vi "modbusRxLoop.vi"(11 "Modbus Port Settings":T1={"Tx Port"="ModbusPort1Tx", "Tx Data FIFO"="txModbusPort1FIFO", "Tx Internal FIFO"="txModbusPort1InternalFIFO", "Tx Telemetry FIFO"="txModbusPort1TelemetryFIFO", "Rx Port"="ModbusPort1Rx", "Rx Data FIFO"="rxModbusPort1FIFO", "Rx Telemetry FIFO"="txModbusPort1TelemetryFIFO", "Base Telemetry Address"=0, "Wait For Rx Frame Register"="WaitForPort1RxFrame", "IRQ Address"=0, "Trigger IRQ Register"="TriggerPort1IRQ", "Trigger IRQ Response Register"="TriggerPort1IRQ"}) -> ()   [LabVIEW 2015]
uses:
  DataTypes/ModbusPortSettings.ctl
  DataTypes/RxLoopData.ctl
  DataTypes/RxStates.ctl
  <vilib>/Platform/TimedLoop/XDataNode/timing_clust.ctl
  <vilib>/Platform/TimedLoop/XDataNode/nitl_modes.ctl
  <vilib>/Platform/TimedLoop/XDataNode/wakeup.ctl
  Telemetry/DataTypes/TelemetryUpdateMode.ctl
  <vilib>/rvi/Emulation/niFpgaSctlEmulationGetInTimedLoop.vi
  <vilib>/rvi/Emulation/niFpgaEmulationReportErrorSimple.vi
  <vilib>/rvi/Emulation/niFpgaGetClockAttributes.vi
  <vilib>/rvi/Emulation/niFpgaCriticalErrorInLSC.vi
  <vilib>/rvi/Emulation/niFpgaEmulationIsFPGAContextNoSignature.vi
  <vilib>/rvi/DataTransferAndStorage/Container/Common/niFpgaContainerGetUniqueNameForEmu.vi
  <vilib>/rvi/Memory/Memory_Emulation/niFpgaMemoryEmulationCacheClearOnFirstRun.vi
  <vilib>/rvi/Memory/Memory_Emulation/nirvimemoryEmulationManagerCache_MakeExclusive.vi
  <vilib>/rvi/Memory/Memory_Emulation/niFpgaMemoryEmulationValidateCache.vi
  <vilib>/rvi/Memory/Memory_Emulation/nirvimemoryEmulationManagerCache_InsertValue.vi
  <vilib>/Utility/error.llb/Clear Errors.vi
  <vilib>/rvi/Memory/Memory_Emulation/nirvimemoryEmulationManagerCache_ReleaseExclusive.vi
  <vilib>/rvi/Memory/Memory_Emulation/nirvimemoryEmulationManagerCache_GetValue.vi
  <vilib>/rvi/Memory/Memory_Emulation/nirvimemoryEmulationManagerCache_SetValue.vi
  <vilib>/rvi/Emulation/niFpgaProcessEmulError.vi
  <vilib>/rvi/eio/common/nirviEmuTemplateMethod_errors.vi
  <vilib>/rvi/DataTransferAndStorage/Container/Common/niFpgaContainerExecOnDevCompGetState.vi
  <vilib>/rvi/errors/niFpgaSetErrorForExecOnDevCompSimple.vi
  <vilib>/rvi/eio/common/nirviEmuReportErrorAndStop.vi
  <vilib>/rvi/FIFO/Fifo_Resource/nirvififoEmulationSetSize.vi
  <vilib>/rvi/FIFO/Fifo_Resource/nirviFifoEmulationQueueMgr.vi
  <instcachedir>/0/nirviFifoEmulationQueueMgr_E5CAEC123FF24DC58D834DCA3CDAA9B5.lvgen/nirviFifoEmulationQueueMgr_E5CAEC123FF24DC58D834DCA3CDAA9B5_005.vi
  <vilib>/rvi/FIFO/Fifo_Resource/nirvififoEmulationDetermineInputValidOut.vi
  <vilib>/rvi/FIFO/Fifo_Resource/nirvififoEmulationCreateLock.vi
  <vilib>/rvi/FIFO/Fifo_Resource/nirvififoEmulationObtainLock.vi
  <vilib>/rvi/FIFO/Fifo_Resource/nirvififoEmulationReleaseLock.vi
  <vilib>/rvi/occurrence/nirviWaitOnOccurrenceBase.vi
  <vilib>/rvi/errors/nirviReportUnexpectedCaseInternalError.vi
  <vilib>/rvi/errors/nirviReportUnexpectedCaseInternalError (U32).vi
  <vilib>/rvi/interface/RandomDataEmulation/niFpgaRandomDataHandleErrors.vi
  <vilib>/Platform/TimedLoop/XDataNode/XDataNode.xnode
  <vilib>/rvi/DataTransferAndStorage/Container/XNode/niFpgaContainer.xnode
  <vilib>/rvi/DataTransferAndStorage/Register/Emulation/niFpgaRegisterEmulation.vi
  <vilib>/eio/EIONode/EIONode.xnode
  <vilib>/rvi/FIFO/Fifo_Resource/niFpgaFifoEmulationRefIn.vi
  <vilib>/rvi/DataTransferAndStorage/Register/Emulation/niFpgaRegisterEmulationRefIn.vi
  <vilib>/Platform/TimedLoop/XDataNode/XDNodeRunTimeDep.lvlib
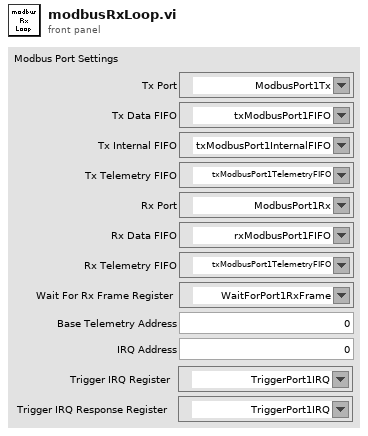
[diagram p1: front panel]
types:
  T1 = typedef "ModbusPortSettings.ctl" = cluster{"Tx Port":refnum<k21>, "Tx Data FIFO":refnum<k21>, "Tx Internal FIFO":refnum<k21>, "Tx Telemetry FIFO":refnum<k21>, "Rx Port":refnum<k21>, "Rx Data FIFO":refnum<k21>, "Rx Telemetry FIFO":refnum<k21>, "Base Telemetry Address":u32, "Wait For Rx Frame Register":refnum<k21>, "IRQ Address":u8, "Trigger IRQ Register":refnum<k21>, "Trigger IRQ Response Register":refnum<k21>}
  T2 = typedef "RxLoopData.ctl" = cluster{"State":T3, "Delay Ticks":u16, "State After Delay":T3, "Number of Samples":u16, "Sample":u8, "Data":u16, "Bits":u16, "State After Insert Sample":T3, "Received Data":bool, "Enqueue Data Time":u32, "Previous Level":bool}
  T3 = typedef "RxStates.ctl" = enum16{"WaitForFallingEdge", "Delay", "SampleStartBit", "SampleBit", "EnqueueData", "EnqueueEndOfFrame"}
  T4 = typedef "XDNodeRunTimeDep.lvlib/timing_clust.ctl" = cluster{"Expected End [f-1]":u64, "Actual End [f-1]":u64, "Finished Late? [f-1]":bool, "Expected End [i-1]":u64, "Actual End [i-1]":u64, "Finished Late? [i-1]":bool, "Expected Start [i]":u64, "Actual Start [i]":u64, "Expected Start [f]":u64, "Actual Start [f]":u64, "Source Name":string, "Structure Name":string, "Period":i64, "Deadline":i64, "Offset":i64, "Start":i64, "Priority":i32, "Timeout":i32, "Mode":T5, "Wakeup Reason":T6, "Error":errorcluster, "Source Type":string, "Secondary Source Type":string, "Global End Time":u64, "Global Start Time":u64, "Frame Duration":u64, "Iteration Duration":u64, "Assigned CPU":i32, "I/O Scan Engine Mode":u32}
  T5 = typedef "XDNodeRunTimeDep.lvlib/nitl_modes.ctl" = enum32{"No Change", "Process missed periods, maintain original phase", "Discard missed periods, maintain original phase", "Process missed periods, ignore original phase", "Discard missed periods, ignore original phase"}
  T6 = typedef "XDNodeRunTimeDep.lvlib/wakeup.ctl" = enum32{"Normal", "Aborted", "Asynchronous wakeup", "Timing source error", "Timed loop error", "Timeout"}
  T7 = typedef "TelemetryUpdateMode.ctl" = enum8{"NOP", "Set", "Add", "Subtract", "Or"}
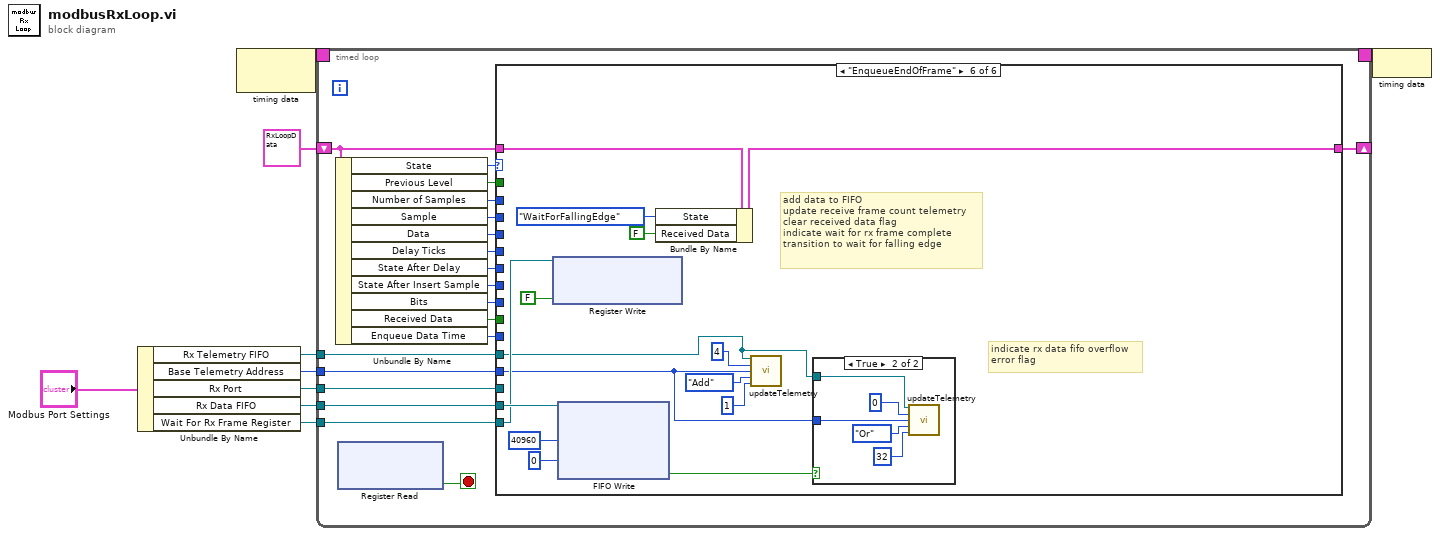
[diagram p0: block diagram]
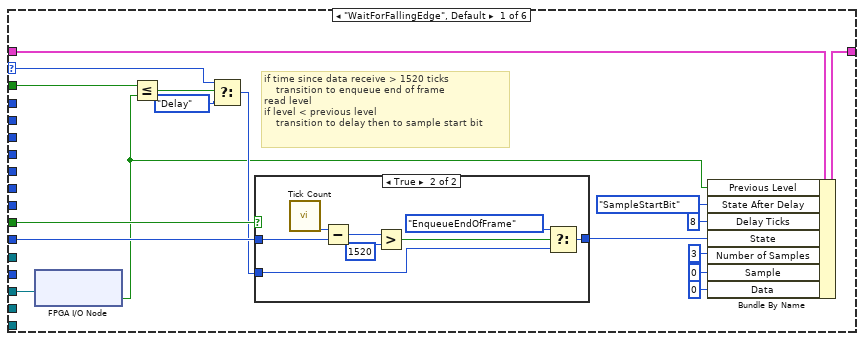
[diagram p2: hidden frame]
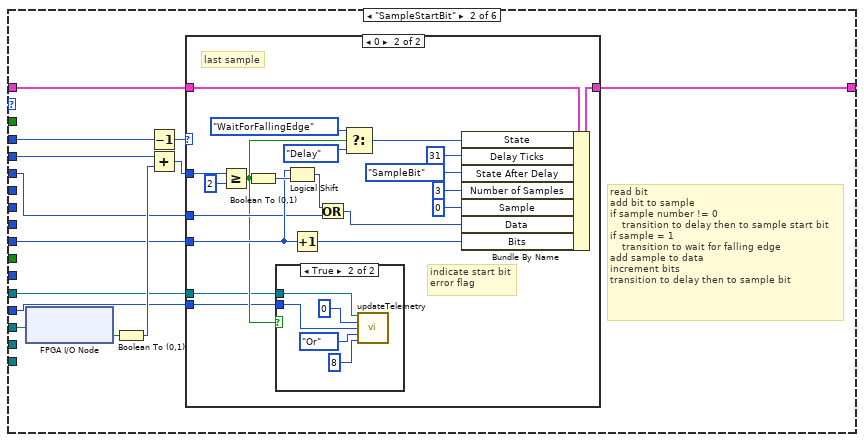
[diagram p4: hidden frame]
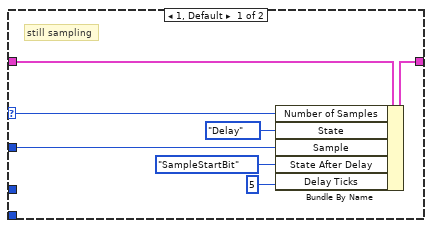
[diagram p5: hidden frame]
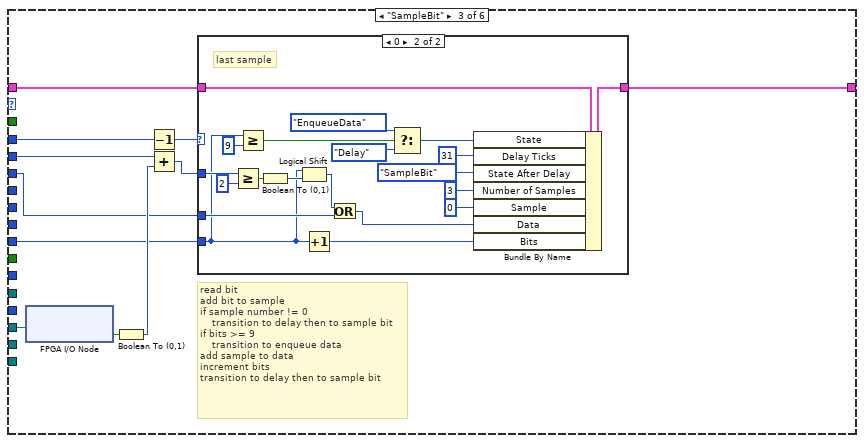
[diagram p7: hidden frame]
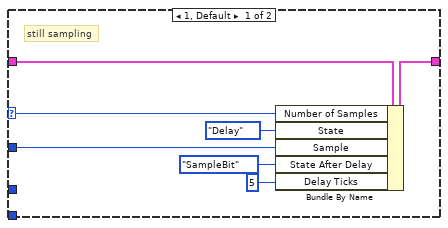
[diagram p8: hidden frame]
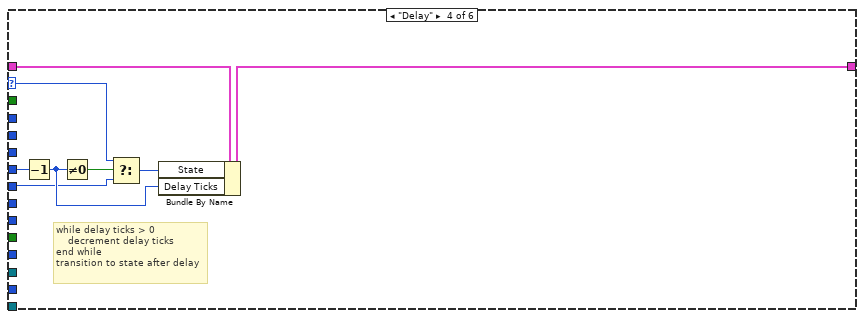
[diagram p9: hidden frame]
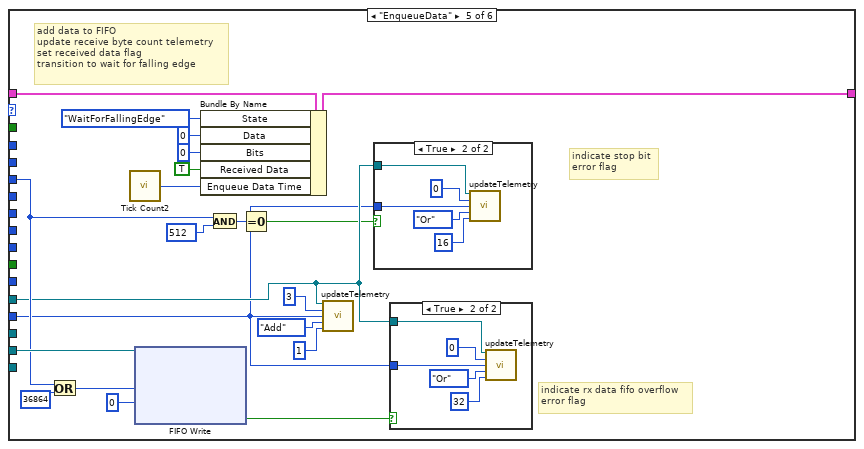
[diagram p10: hidden frame]
diagram:
  n1 = Unbundle By Name("Modbus Port Settings") -> ("Rx Telemetry FIFO"=w6:refnum<k21>, "Base Telemetry Address"=w3:u32, "Rx Port"=w4:refnum<k21>, "Rx Data FIFO"=w5:refnum<k21>, "Wait For Rx Frame Register"=w7:refnum<k21>)
  n2 = node-c288() -> (w9:T4)  [unwired: 1 in]
  n3 = timed-loop {
    tunnel: w4 -> [w25]
    tunnel: w5 -> [w16]
    shift-right: [w24] -> _
    shift-left: T2 {"State"=enum."WaitForFallingEdge", "Delay Ticks"=0, "State After Delay"=enum."WaitForFallingEdge", "Number of Samples"=0, "Sample"=0, "Data"=0, "Bits"=0, "State After Insert Sample"=enum."WaitForFallingEdge", "Received Data"=FALSE, "Enqueue Data Time"=0, "Previous Level"=FALSE} ("ModbusRxLoop") -> [w27]
    tunnel: w3 -> [w13]
    timing: w9 -> [_]
    timing-out: [_] -> w8
    tunnel: w6 -> [w11]
    tunnel: w7 -> [w10]
    stop <- w28 stop-if-true
    n4 = Unbundle By Name(w27) -> ("State"=w26:T3, "Previous Level"=w12:bool, "Number of Samples"=w23:u16, "Sample"=w22:u8, "Data"=w21:u16, "Delay Ticks"=w20:u16, "State After Delay"=w19:T3, "State After Insert Sample"=w18:T3, "Bits"=w17:u16, "Received Data"=w14:bool, "Enqueue Data Time"=w15:u32)
    n5 = xnode ("Register Read")() -> ("Data"=w28:bool)  [unwired: 1 in, 1 out]
    n6 = case shown="\"EnqueueEndOfFrame\"" w26 {
      selector: w26 -> [w44 _ _ w142 _ _]
      tunnel: w27 -> [w38 w62 w105 w139 w165 w188]
      tunnel: w25 -> [w45 w66 w109 _ _ _]
      tunnel: [w41 w61 w104 w138 w164 w185] -> w24
      tunnel: w23 -> [_ w67 w110 _ _ _]
      tunnel: w22 -> [_ w64 w107 _ _ _]
      tunnel: w21 -> [_ w57 w100 _ w151 _]
      tunnel: w20 -> [_ _ _ w140 _ _]
      tunnel: w19 -> [_ _ _ w141 _ _]
      tunnel: w18 -> [_ _ _ _ _ _]
      tunnel: w17 -> [_ w58 w101 _ _ _]
      tunnel: w16 -> [_ _ _ _ w166 w191]
      tunnel: w15 -> [w43 _ _ _ _ _]
      tunnel: w14 -> [w42 _ _ _ _ _]
      tunnel: w13 -> [_ w55 _ _ w147 w179]
      tunnel: w12 -> [w32 _ _ _ _ _]
      tunnel: w11 -> [_ w56 _ _ w148 w178]
      tunnel: w10 -> [_ _ _ _ _ w180]
      frame "WaitForFallingEdge", Default {
        # "if time since data receive > 1520 ticks\n    transition to enqueue end of frame\nread level\nif level < previous level\n    transition to delay then to sample start bit"
        n7 = xnode "FPGA I/O Node"("FPGA I/O In"=w45) -> ("I/O Item"=w29:bool)  [unwired: 1 out]
        n8 = Less Or Equal?(x=w32, y=w29) -> (x <= y?=w35:bool)
        n9 = Select(t=w44, s=w35, f=RxStates."Delay" ("State After Delay")) -> (s? t:f=w34:T3)
        n10 = case shown="True" w42 {
          tunnel: w43 -> [_ w53]
          tunnel: w34 -> [w46 w48]
          tunnel: [w46 w47] -> w39
          frame False {
          }
          frame True {
            n11 = call "Tick Count"() -> ("Tick Count(Ticks)"=w54:u32)
            n12 = Subtract(x=w54, y=w53) -> (x-y=w52:u32)
            n13 = Greater?(x=w52, y=u32 1520) -> (0:w50:bool)
            n14 = Select(t=RxStates."EnqueueEndOfFrame" ("f"), s=w50, f=w48) -> (s? t:f=w47:T3)
          }
        }
        n15 = Bundle By Name(cluster=w38, "Previous Level"=w29, "State After Delay"=RxStates."SampleStartBit", "Delay Ticks"=u16 8 ("Sample"), "State"=w39, "Number of Samples"=u16 3, "Sample"=u8 0, "Data"=u16 0) -> (w41:T2)
      }
      frame "SampleStartBit" {
        # "read bit\nadd bit to sample\nif sample number != 0\n    transition to delay then to sample start bit\nif sample = 1\n    transition to wait for falling edge\nadd sample to data\nincrement bits\ntransition to delay then to sample bit"
        n16 = xnode "FPGA I/O Node"("FPGA I/O In"=w66) -> ("I/O Item"=w65:bool)  [unwired: 1 out]
        n17 = Boolean To (0,1)(Boolean=w65) -> (0, 1=w63:i16)
        n18 = Decrement(x=w67) -> (x-1=w59:u16)
        n19 = Add(x=w64, y=w63) -> (x+y=w60:i16)
        n20 = case shown="0" w59 {
          selector: w59 -> [w71 _]
          tunnel: w60 -> [w72 w92]
          tunnel: w62 -> [w74 w94]
          tunnel: [w73 w93] -> w61
          tunnel: w58 -> [_ w88]
          tunnel: w57 -> [_ w87]
          tunnel: w56 -> [_ w76]
          tunnel: w55 -> [_ w75]
          frame 1, Default {
            # "still sampling"
            n21 = Bundle By Name(cluster=w74, "Number of Samples"=w71, "State"=RxStates."Delay" ("State After Action"), "Sample"=w72, "State After Delay"=RxStates."SampleStartBit", "Delay Ticks"=u16 5) -> (w73:T2)
          }
          frame 0 {
            # "indicate start bit\nerror flag"
            # "last sample"
            n22 = Greater Or Equal?(x=w92, y=i16 2) -> (x >= y?=w77:bool)
            n23 = Boolean To (0,1)(Boolean=w77) -> (0, 1=w89:i16)
            n24 = case shown="True" w77 {
              tunnel: w76 -> [_ w96]
              tunnel: w75 -> [_ w95]
              frame False {
              }
              frame True {
                n25 = call "updateTelemetry.vi"("Telemetry FIFO"=w96, "Address Offset"=u32 0 ("x"), "Base Address"=w95, "Telemetry Update Mode"=TelemetryUpdateMode."Or", "Data"=u32 8) -> ()  [unwired: 11 in]
              }
            }
            n26 = Logical Shift(y=w88, x=w89) -> (x << y=w90:i16)
            n27 = Increment(x=w88) -> (x+1=w86:u16)
            n28 = Or(x=w90, y=w87) -> (x .or. y?=w85:u16)
            n29 = Select(t=RxStates."WaitForFallingEdge", s=w77, f=RxStates."Delay" ("State After Action")) -> (s? t:f=w78:T3)
            n30 = Bundle By Name(cluster=w94, "State"=w78, "Delay Ticks"=u16 31, "State After Delay"=RxStates."SampleBit", "Number of Samples"=u16 3, "Sample"=u8 0, "Data"=w85, "Bits"=w86) -> (w93:T2)
          }
        }
      }
      frame "SampleBit" {
        # "read bit\nadd bit to sample\nif sample number != 0\n    transition to delay then to sample bit\nif bits >= 9\n    transition to enqueue data\nadd sample to data\nincrement bits\ntransition to delay then to sample bit"
        n31 = xnode "FPGA I/O Node"("FPGA I/O In"=w109) -> ("I/O Item"=w108:bool)  [unwired: 1 out]
        n32 = Boolean To (0,1)(Boolean=w108) -> (0, 1=w106:i16)
        n33 = Decrement(x=w110) -> (x-1=w102:u16)
        n34 = Add(x=w107, y=w106) -> (x+y=w103:i16)
        n35 = case shown="0" w102 {
          selector: w102 -> [w114 _]
          tunnel: w103 -> [w115 w135]
          tunnel: w105 -> [w117 w137]
          tunnel: [w116 w136] -> w104
          tunnel: w101 -> [_ w118]
          tunnel: w100 -> [_ w131]
          frame 1, Default {
            # "still sampling"
            n36 = Bundle By Name(cluster=w117, "Number of Samples"=w114, "State"=RxStates."Delay" ("State After Action"), "Sample"=w115, "State After Delay"=RxStates."SampleBit", "Delay Ticks"=u16 5) -> (w116:T2)
          }
          frame 0 {
            # "last sample"
            n37 = Greater Or Equal?(x=w135, y=i16 2) -> (x >= y?=w126:bool)
            n38 = Greater Or Equal?(x=w118, y=u16 9) -> (x >= y?=w119:bool)
            n39 = Boolean To (0,1)(Boolean=w126) -> (0, 1=w132:i16)
            n40 = Logical Shift(y=w118, x=w132) -> (x << y=w133:i16)
            n41 = Increment(x=w118) -> (x+1=w130:u16)
            n42 = Or(x=w133, y=w131) -> (x .or. y?=w129:u16)
            n43 = Select(t=RxStates."EnqueueData", s=w119, f=RxStates."Delay" ("State After Action")) -> (s? t:f=w121:T3)
            n44 = Bundle By Name(cluster=w137, "State"=w121, "Delay Ticks"=u16 31, "State After Delay"=RxStates."SampleBit", "Number of Samples"=u16 3, "Sample"=u8 0, "Data"=w129, "Bits"=w130) -> (w136:T2)
          }
        }
      }
      frame "Delay" {
        # "while delay ticks > 0\n    decrement delay ticks\nend while\ntransition to state after delay"
        n45 = Decrement(x=w140) -> (x-1=w143:u16)
        n46 = Not Equal To 0?(x=w143) -> (x != 0?=w145:bool)
        n47 = Select(t=w142, s=w145, f=w141) -> (s? t:f=w144:T3)
        n48 = Bundle By Name(cluster=w139, "State"=w144, "Delay Ticks"=w143) -> (w138:T2)
      }
      frame "EnqueueData" {
        # "indicate stop bit\nerror flag"
        # "indicate rx data fifo overflow\nerror flag"
        # "add data to FIFO\nupdate receive byte count telemetry\nset received data flag\ntransition to wait for falling edge"
        n49 = Or(x=w151, y=u16 36864 ("Data")) -> (x .or. y?=w157:u16)
        n50 = call "Tick Count2"() -> ("Tick Count(Ticks)"=w161:u32)
        n51 = xnode ("FIFO Write")("Element"=w157, "Timeout"=0, "FIFO In"=w166) -> ("Timed Out?"=w152:bool)  [unwired: 1 out]
        n52 = Bundle By Name(cluster=w165, "State"=RxStates."WaitForFallingEdge", "Data"=u16 0, "Bits"=u16 0, "Received Data"=TRUE, "Enqueue Data Time"=w161) -> (w164:T2)
        n53 = And(x=w151, y=u16 512 ("Data")) -> (x .and. y?=w149:u16)
        n54 = Equal To 0?(x=w149) -> (x = 0?=w146:bool)
        n55 = call "updateTelemetry.vi"("Telemetry FIFO"=w148, "Address Offset"=u32 3 ("x"), "Base Address"=w147, "Telemetry Update Mode"=TelemetryUpdateMode."Add", "Data"=u32 1) -> ()  [unwired: 11 in]
        n56 = case shown="True" w146 {
          tunnel: w148 -> [_ w168]
          tunnel: w147 -> [_ w167]
          frame False {
          }
          frame True {
            n57 = call "updateTelemetry.vi"("Telemetry FIFO"=w168, "Address Offset"=u32 0 ("x"), "Base Address"=w167, "Telemetry Update Mode"=TelemetryUpdateMode."Or", "Data"=u32 16) -> ()  [unwired: 11 in]
          }
        }
        n58 = case shown="True" w152 {
          tunnel: w148 -> [_ w173]
          tunnel: w147 -> [_ w172]
          frame False {
          }
          frame True {
            n59 = call "updateTelemetry.vi"("Telemetry FIFO"=w173, "Address Offset"=u32 0 ("x"), "Base Address"=w172, "Telemetry Update Mode"=TelemetryUpdateMode."Or", "Data"=u32 32) -> ()  [unwired: 11 in]
          }
        }
      }
      frame "EnqueueEndOfFrame" {
        # "indicate rx data fifo overflow\nerror flag"
        # "add data to FIFO\nupdate receive frame count telemetry\nclear received data flag\nindicate wait for rx frame complete\ntransition to wait for falling edge"
        n60 = xnode ("Register Write")("Data"=FALSE, "Register In"=w180) -> ()  [unwired: 1 out]
        n61 = xnode ("FIFO Write")("Element"=u16 40960, "Timeout"=0, "FIFO In"=w191) -> ("Timed Out?"=w177:bool)  [unwired: 1 out]
        n62 = Bundle By Name(cluster=w188, "State"=RxStates."WaitForFallingEdge", "Received Data"=FALSE) -> (w185:T2)
        n63 = call "updateTelemetry.vi"("Telemetry FIFO"=w178, "Address Offset"=u32 4 ("x"), "Base Address"=w179, "Telemetry Update Mode"=TelemetryUpdateMode."Add", "Data"=u32 1) -> ()  [unwired: 11 in]
        n64 = case shown="True" w177 {
          tunnel: w178 -> [_ w193]
          tunnel: w179 -> [_ w192]
          frame False {
          }
          frame True {
            n65 = call "updateTelemetry.vi"("Telemetry FIFO"=w193, "Address Offset"=u32 0 ("x"), "Base Address"=w192, "Telemetry Update Mode"=TelemetryUpdateMode."Or", "Data"=u32 32) -> ()  [unwired: 11 in]
          }
        }
      }
    }
  }
  n66 = node-c288(w8) -> ()
